vi "Convert_pick-place_line.vi"(11 "sequence line":string[](array[string])) -> (3 "command":string[](array[string]))   [LabVIEW 2017]
panel:
  in  "ダミー":string[](array[string])
  out "文字列":string
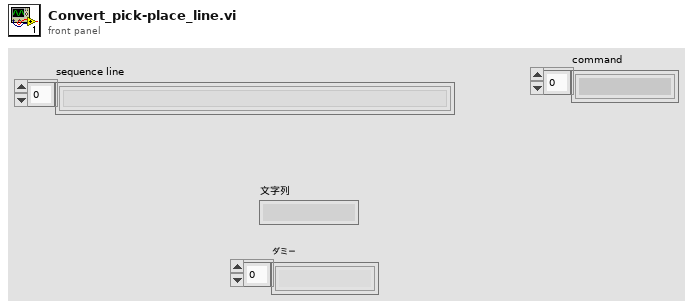
[diagram p1: front panel]
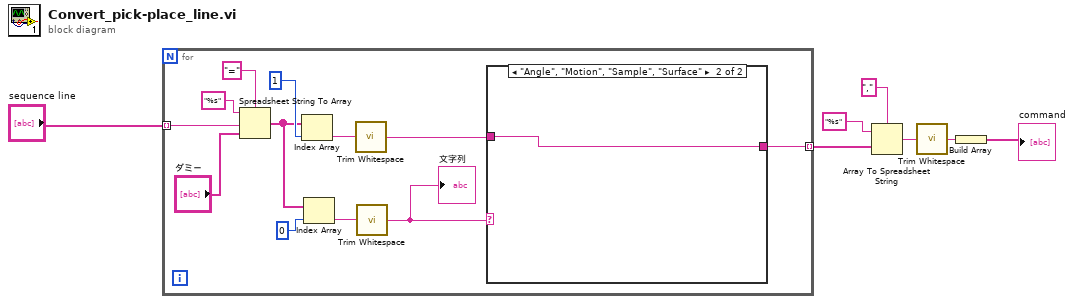
[diagram p0: block diagram]
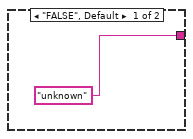
[diagram p2: hidden frame]
diagram:
  n1 = for {
    tunnel: "sequence line" -> [w19] mode=indexing
    tunnel: [w12] -> w7 mode=indexing
    n2 = Spreadsheet String To Array(delimiter (Tab)="=", format string="%s", spreadsheet string=w19, array type (2D Dbl)="ダミー") -> (array=w14:string[])
    n3 = Index Array(array=w14, index=1) -> (element=w10:string)
    n4 = Index Array(array=w14, index=0) -> (element=w11:string)
    n5 = call <vilib>:"Trim Whitespace.vi"("string"=w10) -> ("trimmed string"=w9:string)  [unwired: 1 in]
    n6 = call <vilib>:"Trim Whitespace.vi"("string"=w11) -> ("trimmed string"=w8:string)  [unwired: 1 in]
    "文字列" <- w8
    n7 = case shown="\"Angle\", \"Motion\", \"Sample\", \"Surface\"" w8 {
      tunnel: w9 -> [_ w21]
      tunnel: ["unknown" w21] -> w12
      frame "FALSE", Default {
      }
      frame "Angle", "Motion", "Sample", "Surface" {
      }
    }
  }
  n8 = Array To Spreadsheet String(delimiter (Tab)=",", array=w7, 3:"%s") -> (spreadsheet string=w1:string)
  n9 = call <vilib>:"Trim Whitespace.vi"("string"=w1) -> ("trimmed string"=w2:string)  [unwired: 1 in]
  n10 = Build Array(w2) -> (→"command":string[])
